vi "DecrementIfNotZero.vi"(1 "Input":dbl) -> (0 "Decremented Value":dbl)   [LabVIEW 2014]
doc: "This VI will decrement the input by one. If the input is a double greater than one, it will it will output one minus the input. if the input is less than one, but greater than zero, it will replace the value with zero. If the input is zero, the output will also be zero."
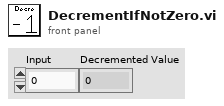
[diagram p1: front panel]
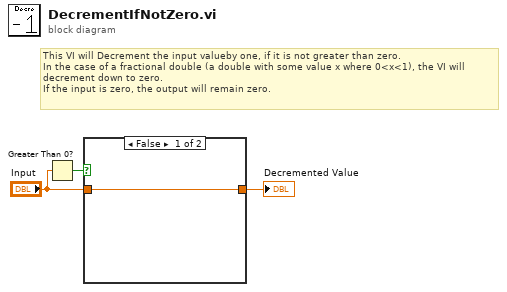
[diagram p0: block diagram]
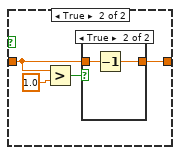
[diagram p2: hidden frame]
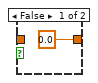
[diagram p3: hidden frame]
diagram:
  # "This VI will Decrement the input valueby one, if it is not greater than zero. \nIn the case of a fractional double (a double with some value x where 0<x<1), the VI will\ndecrement down to zero.\nIf the input is zero, the output will remain zero."
  n1 = Greater Than 0?(x="Input") -> (x > 0?=w3:bool)
  n2 = case shown="False" w3 {
    tunnel: "Input" -> [w4 w7]
    tunnel: [w4 w5] -> w1
    frame False {
    }
    frame True {
      n3 = Greater?(x=w7, y=1.0) -> (0:w8:bool)
      n4 = case shown="True" w8 {
        tunnel: w7 -> [_ w11]
        tunnel: [0.0 w10] -> w5
        frame False {
        }
        frame True {
          n5 = Decrement(x=w11) -> (x-1=w10:dbl)
        }
      }
    }
  }
  "Decremented Value" <- w1
